vi "Write to String Log.vi"(10 "Log Entry":string, 11 "String Control Sink in":refnum<class "String Control Sink.lvclass">) -> (0 "error out":errorcluster, 3 "String Control Sink out":refnum<class "String Control Sink.lvclass">)   [LabVIEW 2019, in "String Control Sink.lvclass"]
uses:
  String Control Sink.lvclass
  String Control Sink.lvclass/String Control Sink.ctl
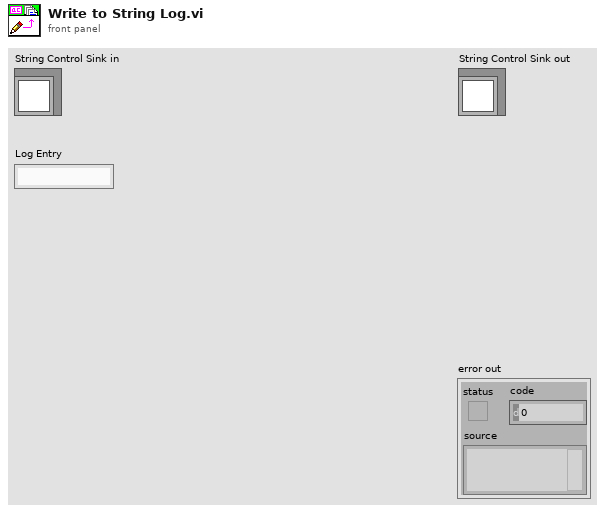
[diagram p1: front panel]
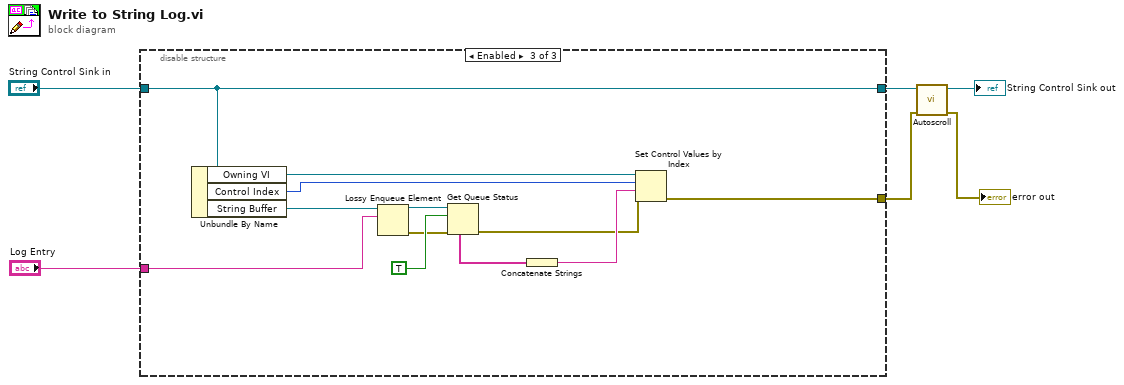
[diagram p0: block diagram]
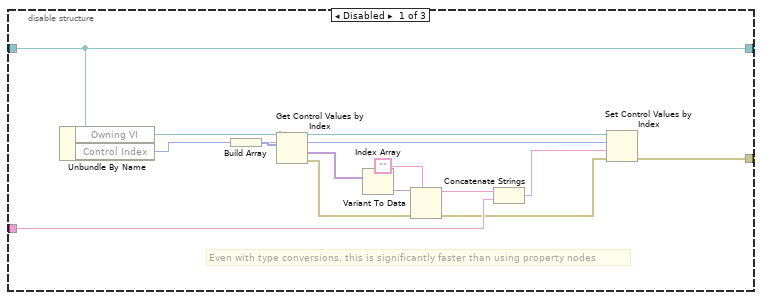
[diagram p2: hidden frame]
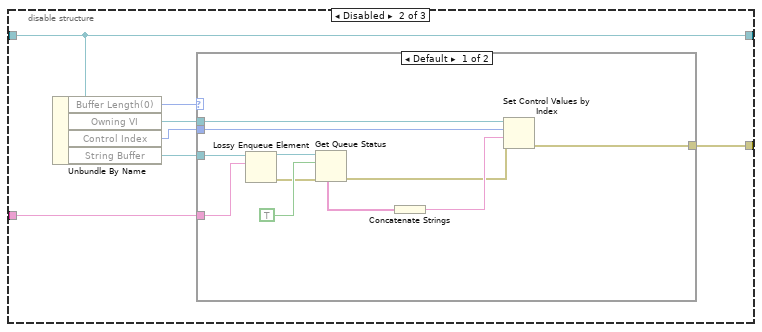
[diagram p3: hidden frame]
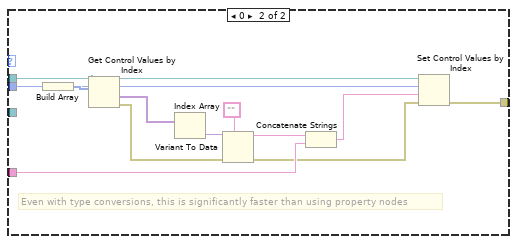
[diagram p4: hidden frame]
diagram:
  n1 = disable-structure shown="Enabled" {
    disable-tunnel: "Log Entry" -> [w15 w26 w61]
    disable-tunnel: "String Control Sink in" -> [w7 w22 w57]
    disable-tunnel: [w8 w23 w58] -> w3
    disable-tunnel: [w7 w22 w57] -> w1
    frame Disabled {
      # "Even with type conversions, this is significantly faster than using property nodes"
      n2 = Unbundle By Name(w7) -> ("Owning VI"=w12:refnum<vi>, "Control Index"=w9:i32)
      n3 = Build Array(w9) -> (w11:i32[])
      n4 = Get Control Values by Index(0:w12, 1:w11) -> (10:w19:variant[], 11:w14:errorcluster)  [unwired: 1 in]
      n5 = Index Array(array=w19) -> (element=w18:variant)  [unwired: 1 in]
      n6 = Variant To Data(error in=w14, type="", Variant=w18) -> (data=w16:string, error out=w13:errorcluster)
      n7 = Concatenate Strings(w16, w15) -> (w10:string)
      n8 = Set Control Values by Index(0:w12, 1:w9, 2:w10, 3:w13) -> (11:w8:errorcluster)
    }
    frame Disabled {
      n9 = Unbundle By Name(w22) -> ("Buffer Length(0)"=w21:i32, "Owning VI"=w25:refnum<vi>, "Control Index"=w24:i32, "String Buffer"=w20:refnum<queue>)
      n10 = case shown="Default" w21 {
        tunnel: w26 -> [w36 w45]
        tunnel: w25 -> [w33 w42]
        tunnel: w24 -> [w32 w39]
        tunnel: [w27 w38] -> w23
        tunnel: w20 -> [w37 _]
        frame Default {
          n11 = Lossy Enqueue Element(queue=w37, element=w36) -> (queue out=w35:refnum<queue>, error out=w31:errorcluster)  [unwired: 1 in, 2 out]
          n12 = Get Queue Status(queue=w35, return elements? (F)=TRUE, error in (no error)=w31) -> (error out=w28:errorcluster, elements=w30:string[])  [unwired: 6 out]
          n13 = Concatenate Strings(w30) -> (w29:string)
          n14 = Set Control Values by Index(0:w33, 1:w32, 2:w29, 3:w28) -> (11:w27:errorcluster)
        }
        frame 0 {
          # "Even with type conversions, this is significantly faster than using property nodes"
          n15 = Build Array(w39) -> (w41:i32[])
          n16 = Get Control Values by Index(0:w42, 1:w41) -> (10:w49:variant[], 11:w44:errorcluster)  [unwired: 1 in]
          n17 = Index Array(array=w49) -> (element=w48:variant)  [unwired: 1 in]
          n18 = Variant To Data(error in=w44, type="", Variant=w48) -> (data=w46:string, error out=w43:errorcluster)
          n19 = Concatenate Strings(w46, w45) -> (w40:string)
          n20 = Set Control Values by Index(0:w42, 1:w39, 2:w40, 3:w43) -> (11:w38:errorcluster)
        }
      }
    }
    frame Enabled {
      n21 = Unbundle By Name(w57) -> ("Owning VI"=w60:refnum<vi>, "Control Index"=w59:i32, "String Buffer"=w56:refnum<queue>)
      n22 = Lossy Enqueue Element(queue=w56, element=w61) -> (queue out=w55:refnum<queue>, error out=w53:errorcluster)  [unwired: 1 in, 2 out]
      n23 = Get Queue Status(queue=w55, return elements? (F)=TRUE, error in (no error)=w53) -> (error out=w50:errorcluster, elements=w52:string[])  [unwired: 6 out]
      n24 = Concatenate Strings(w52) -> (w51:string)
      n25 = Set Control Values by Index(0:w60, 1:w59, 2:w51, 3:w50) -> (11:w58:errorcluster)
    }
  }
  n26 = call "Autoscroll.vi"("error in (no error)"=w3, "String Control Sink in"=w1) -> ("error out"=→"error out":errorcluster, "String Control Sink out"=→"String Control Sink out":refnum<class "String Control Sink.lvclass">)  [unwired: 8 in]
